vi "Image-binarization.vi"(8 "error in":errorcluster, 10 "Buffer element in":T1 {"Temperature characteristics"."Stand. dev. temperature" format="%#.1f"; "Temperature characteristics"."Min. temperature" format="%#.0f"; "Temperature characteristics"."Max. temperature" format="%#.0f"; "Temperature characteristics"."Average temperature" format="%#.0f"}, 11 "Analysis params. ref. in":refnum<data-value>) -> (0 "error IO":errorcluster, 2 "Buffer element":T1 {"Temperature characteristics"."Stand. dev. temperature" format="%#.1f"; "Temperature characteristics"."Min. temperature" format="%#.0f"; "Temperature characteristics"."Max. temperature" format="%#.0f"; "Temperature characteristics"."Average temperature" format="%#.0f"}, 3 "Analysis params. ref.":refnum<data-value>)   [LabVIEW 2013, in "CameraVision.lvlib" / "CV-Main.lvclass"]
uses:
  CV-Main.lvclass
  Analysis/CV-Analysis.lvclass
  Buffers/Storage-buffer.ctl
  <vilib>/vision/Image Controls.llb/IMAQ Image.ctl
  Temperature/Temperature-characteristics.ctl
  Analysis/Characteristics-cluster.ctl
  Analysis/CV-Analysis.lvclass/CV-Analysis.ctl
  Analysis/Read Melt-pool characteristics.vi
  Analysis/Read Binarization treshold.vi
  <vilib>/vision/NI_Vision_Development_Module.lvlib
  Temperature/CV-Temperature.lvclass
  Buffers/CV-Buffers.lvclass
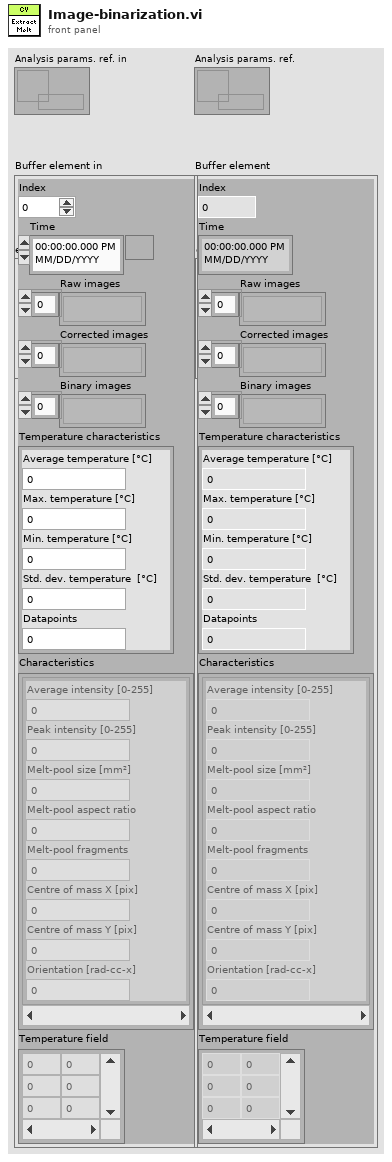
[diagram p1: front panel]
types:
  T1 = typedef "CameraVision.lvlib/CV-Buffers.lvclass/Storage-buffer.ctl" = cluster{"Index":i32, "Time":timestamp, "Raw images":T2[], "Corrected images":T2[], "Binary images":T2[], "Temperature characteristics":T3, "Characteristics":T4[], "Temperature field":dbl[][]}
  T2 = typedef "IMAQ Image.ctl" = refnum<image>
  T3 = typedef "CameraVision.lvlib/CV-Temperature.lvclass/Temperature-characteristics.ctl" = cluster{"Average temperature ":dbl, "Max. temperature":dbl, "Min. temperature":dbl, "Stand. dev. temperature":dbl, "Datapoints":dbl}
  T4 = typedef "CameraVision.lvlib/CV-Analysis.lvclass/Characteristics-cluster.ctl" = cluster{"Average intensity":dbl, "Peak intensity":dbl, "Melt-pool size":dbl, "Melt-pool aspect ratio":dbl, "Melt-pool fragments":dbl, "Centre of mass X":dbl, "Centre of mass Y":dbl, "Orientation":dbl}
  T5 = cluster{"Accessors RO:Binarization treshold":sgl, sgl}
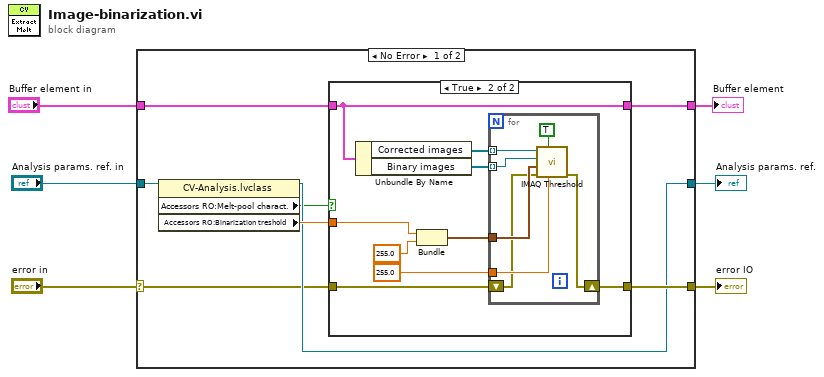
[diagram p0: block diagram]
diagram:
  n1 = case shown="No Error" "error in" {
    selector: "error in" -> [w7 w35]
    tunnel: [w13 w35] -> w5
    tunnel: "Buffer element in" -> [w14 w33]
    tunnel: "Analysis params. ref. in" -> [w12 w34]
    tunnel: [w10 w34] -> w2
    tunnel: [w9 w33] -> w1
    frame No Error {
      n2 = property class="CV-Analysis.lvclass"(reference=w12) -> (reference out=w10:refnum<data-value>, "Accessors RO:Melt-pool charact."=w8:bool, "Accessors RO:Binarization treshold"=w11:sgl)  [unwired: 1 in, 1 out]
      n3 = case shown="True" w8 {
        tunnel: w14 -> [w15 w17]
        tunnel: w11 -> [_ w18]
        tunnel: w7 -> [w16 w20]
        tunnel: [w16 w19] -> w13
        tunnel: [w15 w17] -> w9
        frame False {
        }
        frame True {
          n4 = Unbundle By Name(w17) -> ("Corrected images"=w25:T2[], "Binary images"=w24:T2[])
          n5 = Bundle("Accessors RO:Binarization treshold"=w18, sgl 255.0) -> (w21:T5)  [unwired: 1 in]
          n6 = for {
            tunnel: w25 -> [w32] mode=indexing
            tunnel: w24 -> [w31] mode=indexing
            tunnel: sgl 255.0 -> [w30]
            tunnel: w21 -> [w29]
            shift-right: [w27] -> w19
            shift-left: w20 -> [w28]
            n7 = call "IMAQ Threshold"("Replace Value"=w30, "Keep/Replace Value (Replace)"=TRUE, "error in (no error)"=w28, "Range"=w29, "Image Dst"=w31, "Image Src"=w32) -> ("error out"=w27:errorcluster)  [unwired: 4 in, 1 out]
          }
        }
      }
    }
    frame Error {
    }
  }
  "error IO" <- w5
  "Buffer element" <- w1
  "Analysis params. ref." <- w2
